vi "ATF-Storage Device List.vi"(9 "DL":string, 11 "Enum":enum16{"Read", "Write", "Clear"}(ring)) -> (1 "DL":string)   [LabVIEW 2022 SP3]
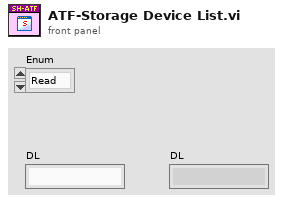
[diagram p1: front panel]
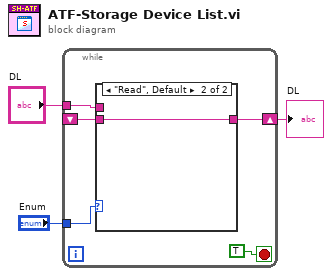
[diagram p0: block diagram]
diagram:
  n1 = while {
    tunnel: "Enum" -> [w8]
    tunnel: "DL" -> [w7]
    shift-right: [w6] -> w1
    shift-left: _ -> [w5]
    stop <- TRUE stop-if-true
    n2 = case shown="\"Read\", Default" w8 {
      tunnel: w7 -> [w9 _]
      tunnel: [w9 w10] -> w6
      tunnel: w5 -> [_ w10]
      frame "Write" {
      }
      frame "Read", Default {
      }
    }
  }
  "DL" <- w1
